vi "circle_target.vi"(8 "y0":dbl, 9 "x0":dbl, 11 "Target's width":i32) -> (1 "Target plots":cluster{dbl[], dbl[]}[](array[cluster]), 3 "Target pixels":cluster{dbl[], dbl[]})   [LabVIEW 2010]
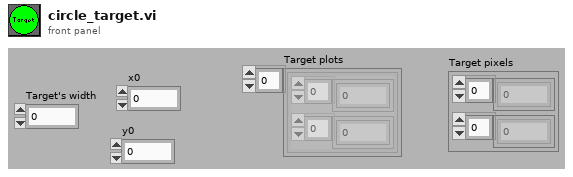
[diagram p1: front panel]
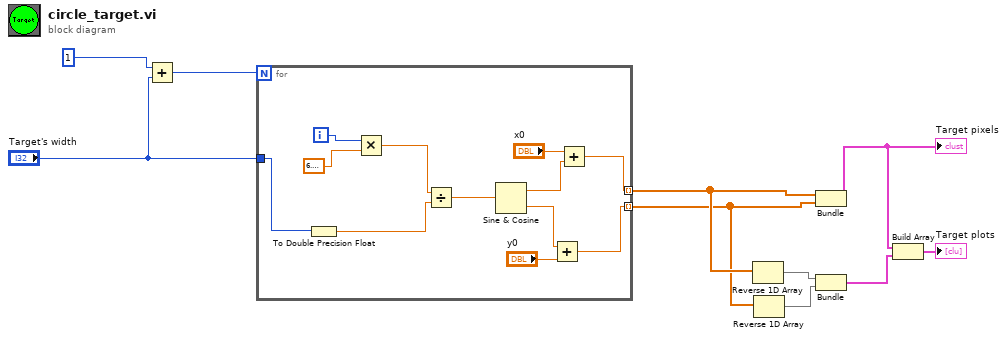
[diagram p0: block diagram]
diagram:
  n1 = Add(x=1 ("y"), y="Target's width") -> (x+y=w10:i32)
  n2 = for {
    N: w10 -> [_]
    tunnel: [w16] -> w6 mode=indexing
    tunnel: [w15] -> w5 mode=indexing
    tunnel: "Target's width" -> [w14]
    i -> [w22]
    n3 = To Double Precision Float(number=w14) -> (double precision float=w13:dbl)
    n4 = Multiply(x=w22, y=6.283185307179586) -> (x*y=w20:dbl)
    n5 = Divide(x=w20, y=w13) -> (x/y=w19:dbl)
    n6 = Sine & Cosine(0:w19) -> (1:w18:dbl, 2:w17:dbl)
    n7 = Add(x=w17, y="y0") -> (x+y=w15:dbl)
    n8 = Add(x="x0", y=w18) -> (x+y=w16:dbl)
  }
  n9 = Reverse 1D Array(array=w6) -> (reversed array=w4:dbl[])
  n10 = Reverse 1D Array(array=w5) -> (reversed array=w3:dbl[])
  n11 = Bundle(w6, w5) -> (w7:cluster{dbl[], dbl[]})  [unwired: 1 in]
  "Target pixels" <- w7
  n12 = Bundle(w4, w3) -> (w2:cluster{dbl[], dbl[]})  [unwired: 1 in]
  n13 = Build Array(w7, w2) -> (→"Target plots":cluster{dbl[], dbl[]}[])
